vi "List All Shared Variables.vi"(8 "error in":errorcluster) -> (0 "error out":errorcluster, 2 "Variable Descriptions":T1[](array[typedef]), 3 "Variable References":refnum<k21>[](array[refnum]))   [LabVIEW 2017, in "Shared Variables Library.lvlib"]
doc: "Get a list and description of all local shared variables."
uses:
  Shared Variables Library.lvlib
  Typedefs/Shared Variable Properties--Cluster.ctl
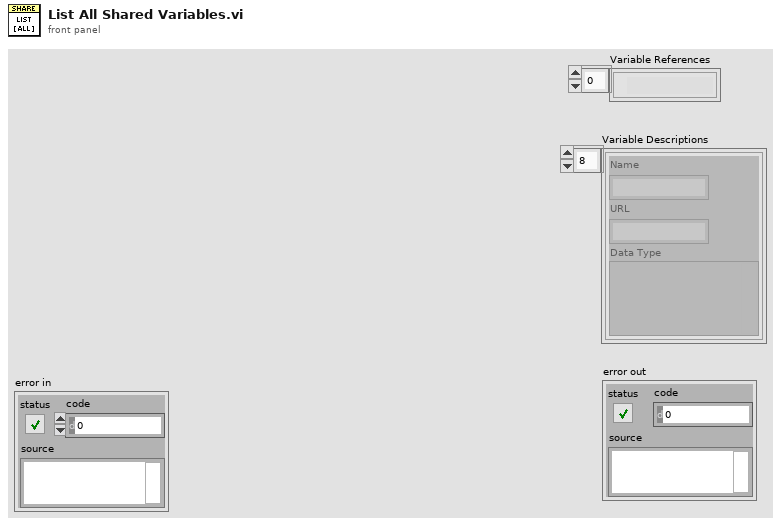
[diagram p1: front panel]
types:
  T1 = typedef "Shared Variables Library.lvlib/Shared Variable Properties--Cluster.ctl" = cluster{"Name":string, "URL":string, "Data Type":variant}
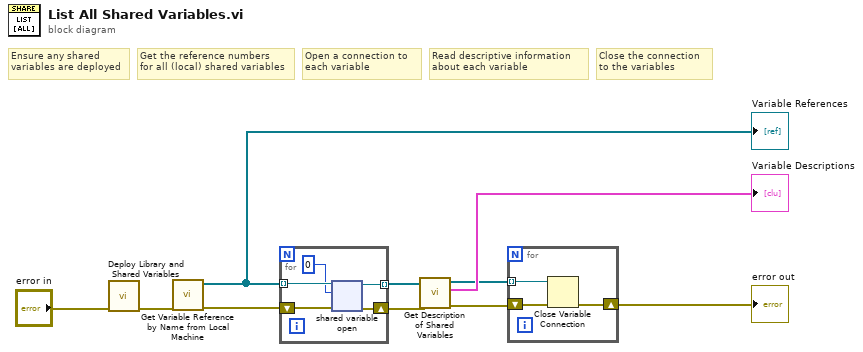
[diagram p0: block diagram]
diagram:
  # "Close the connection\nto the variables"
  # "Read descriptive information \nabout each variable"
  # "Open a connection to\neach variable"
  # "Get the reference numbers\nfor all (local) shared variables"
  # "Ensure any shared\nvariables are deployed"
  n1 = call "Deploy Library and Shared Variables.vi"("error in"="error in") -> ("error out"=w9:errorcluster)  [unwired: 10 in]
  n2 = call "Get Variable Reference by Name from Local Machine.vi"("error in"=w9) -> ("error out"=w4:errorcluster, "Variable References Out"=w2:refnum<k21>[])  [unwired: 8 in, 1 out]
  "Variable References" <- w2
  n3 = for {
    shift-right: [w14] -> w3
    shift-left: w4 -> [w15]
    tunnel: w2 -> [w13] mode=indexing
    tunnel: [w11] -> w1 mode=indexing
    n4 = shared-variable-open(w13, w15, i16 0) -> (w11:refnum<k21>, w14:errorcluster)  [unwired: 1 in]
  }
  n5 = call "Get Description of Shared Variables.vi"("error in"=w3, "Variable References In"=w1) -> ("error out"=w6:errorcluster, "Variable Descriptions"=→"Variable Descriptions":T1[], "Variable References Out"=w5:refnum<k21>[])  [unwired: 7 in]
  n6 = for {
    shift-right: [w16] -> w8
    shift-left: w6 -> [w18]
    tunnel: w5 -> [w17] mode=indexing
    n7 = Close Variable Connection(8:w18, 11:w17) -> (0:w16:errorcluster)
  }
  "error out" <- w8
